vi "Application Data Folder.vi"(8 "error in (no error)":errorcluster) -> (0 "error out":errorcluster, 1 "Config Filepath":path, 2 "Error Logs Folder":path, 3 "Application Data Folder":path, 4 "Campaign Folder":path)   [LabVIEW 2018, in "Config Module.lvlib"]
uses:
  Config Module.lvlib
  <vilib>/Utility/sysdir.llb/System Directory Type.ctl
  Utilities/Utilities 1.lvlib
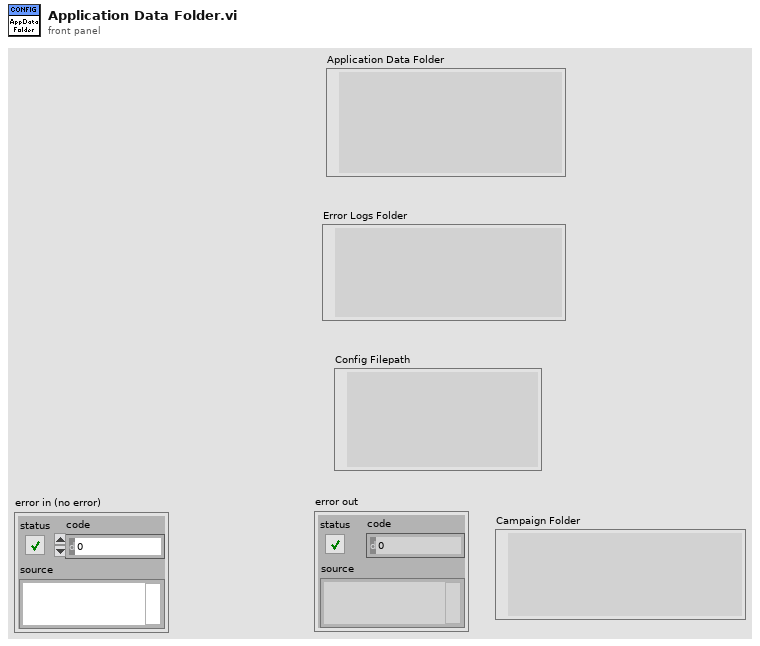
[diagram p1: front panel]
types:
  T1 = typedef "System Directory Type.ctl" = i32
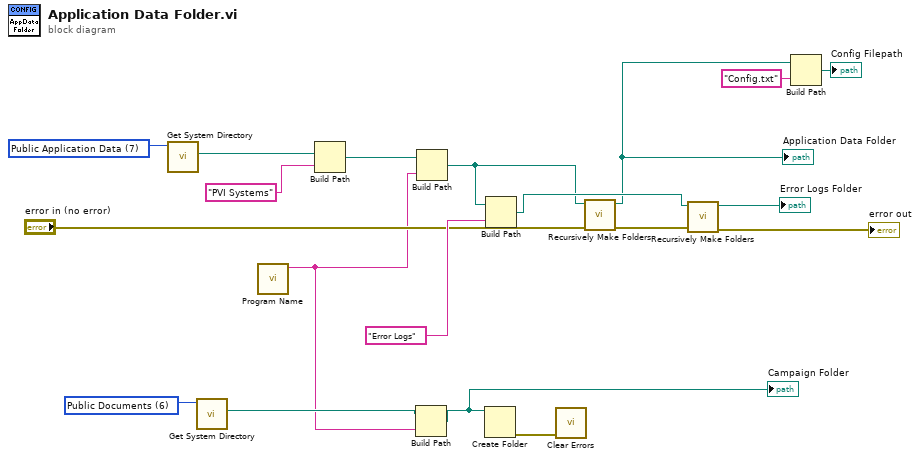
[diagram p0: block diagram]
diagram:
  w5 = T1 6 items=["User Home"=0, "User Desktop"=1, "User Documents"=2, "User Application Data"=3, "User Preferences"=4, "User Temporary"=5, "Public Documents"=6, "Public Application Data"=7, "Public Preferences"=8, "Public Cache"=13, "System Core Libraries"=9, "System Installed Libraries"=10, "Application Files"=11, "Boot Volume Root"=12] ("system directory type")
  w19 = T1 7 items=["User Home"=0, "User Desktop"=1, "User Documents"=2, "User Application Data"=3, "User Preferences"=4, "User Temporary"=5, "Public Documents"=6, "Public Application Data"=7, "Public Preferences"=8, "Public Cache"=13, "System Core Libraries"=9, "System Installed Libraries"=10, "Application Files"=11, "Boot Volume Root"=12] ("system directory type")
  n1 = call <vilib>:"Get System Directory.vi"("system directory type"=w19) -> ("system directory"=w18:path)  [unwired: 10 in]
  n2 = call <vilib>:"Get System Directory.vi"("system directory type"=w5) -> ("system directory"=w4:path)  [unwired: 10 in]
  n3 = call "Program Name.vi"() -> ("Program Name"=w3:string)  [unwired: 11 in]
  n4 = Build Path(base path=w18, name or relative path="PVI Systems") -> (appended path=w15:path)
  n5 = Build Path(base path=w4, name or relative path=w3) -> (appended path=w2:path)
  "Campaign Folder" <- w2
  n6 = Build Path(base path=w15, name or relative path=w3) -> (appended path=w10:path)
  n7 = Create Folder(path (use dialog)=w2) -> (error out=w1:errorcluster)  [unwired: 2 in, 2 out]
  n8 = Build Path(base path=w10, name or relative path="Error Logs") -> (appended path=w14:path)
  n9 = call <vilib>:"Clear Errors.vi"("error in (no error)"=w1) -> ()  [unwired: 5 in, 2 out]
  n10 = call "Recursively Make Folders.vi"("error in (no error)"="error in (no error)", "directory path"=w10) -> ("error out"=w12:errorcluster, "directory path 2"=w7:path)  [unwired: 4 in]
  "Application Data Folder" <- w7
  n11 = call "Recursively Make Folders.vi"("error in (no error)"=w12, "directory path"=w14) -> ("error out"=→"error out":errorcluster, "directory path 2"=→"Error Logs Folder":path)  [unwired: 4 in]
  n12 = Build Path(base path=w7, name or relative path="Config.txt") -> (appended path=→"Config Filepath":path)
